vi "Voltage_demand.vi"() -> ()   [LabVIEW 2013]
uses:
  <vilib>/DAQmx/create/channels.llb/DAQmx Create Channel (CO-Pulse Generation-Frequency).vi
  <vilib>/DAQmx/configure/timing.llb/DAQmx Timing (Implicit).vi
panel:
  in  "stop vi":bool
  in  "counter":tag
  in  "stop blinking":bool
  in  "Blink":bool
  in  "Frequency [Hz]":dbl format="%#_3p"
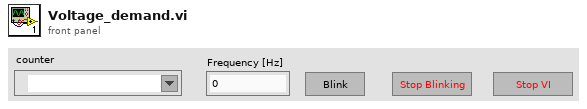
[diagram p1: front panel]
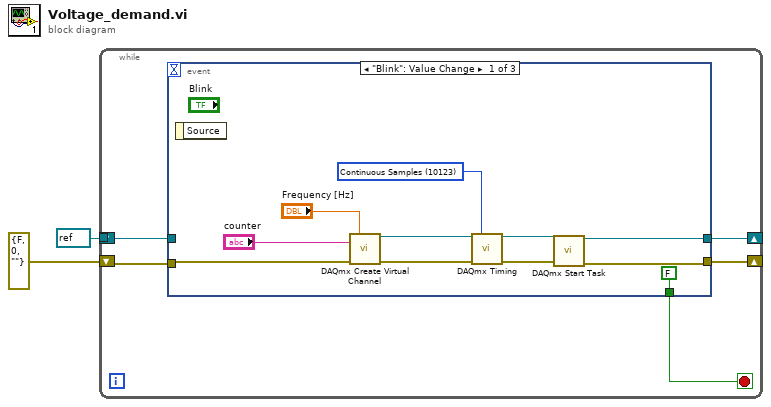
[diagram p0: block diagram]
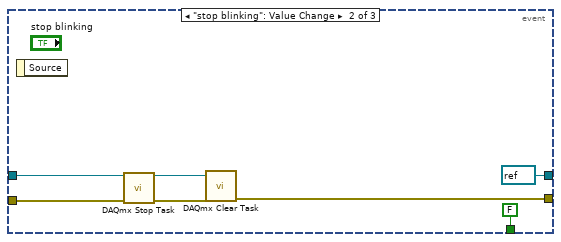
[diagram p2: hidden frame]
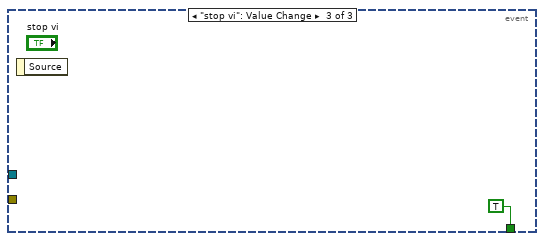
[diagram p3: hidden frame]
diagram:
  n1 = while {
    shift-right: [w6] -> _
    shift-left: refnum<k21> refnum ("task out") -> [w7]
    tunnel: [w7] -> _
    shift-right: [w4] -> _
    shift-left: errorcluster {"status"=FALSE, "code"=0, "source"=""} ("error out") -> [w5]
    stop <- w3 stop-if-true
    n2 = event shown="[0] \"Blink\": Value Change" {
      selector: _ -> [_ _ _]
      dyn-events: _ -> [_ _ _]
      timeout: _ -> [_ _ _]
      tunnel: [w11 refnum<k21> refnum ("task out") _] -> w6
      tunnel: w7 -> [_ w25 _]
      tunnel: w5 -> [w10 w23 _]
      tunnel: [w9 w22 _] -> w4
      tunnel: [FALSE FALSE TRUE] -> w3
      event "Blink": Value Change {
        w14 = 10123 items=["Finite Samples"=10178, "Continuous Samples"=10123, "Hardware Timed Single Point"=12522] ("sample mode")
        n3 = event-data() -> ()  [unwired: 1 in, 1 out]
        n4 = call-poly <vilib>:"DAQmx Create Virtual Channel.vi"("frequency"="Frequency [Hz]", "counter"="counter", "error in"=w10) -> ("task out"=w16:refnum<k21>, "error out"=w15:errorcluster)  [unwired: 11 in]
        n5 = call-poly <vilib>:"DAQmx Timing.vi"("task/channels in"=w16, "sample mode"=w14, "error in"=w15) -> ("task out"=w13:refnum<k21>, "error out"=w12:errorcluster)  [unwired: 11 in]
        n6 = call <vilib>:"DAQmx Start Task.vi"("task/channels in"=w13, "error in"=w12) -> ("task out"=w11:refnum<k21>, "error out"=w9:errorcluster)  [unwired: 12 in]
      }
      event "stop blinking": Value Change {
        n7 = event-data() -> ()  [unwired: 1 in, 1 out]
        n8 = call <vilib>:"DAQmx Stop Task.vi"("task/channels in"=w25, "error in"=w23) -> ("task out"=w24:refnum<k21>, "error out"=w21:errorcluster)  [unwired: 12 in]
        n9 = call <vilib>:"DAQmx Clear Task.vi"("task in"=w24, "error in"=w21) -> ("error out"=w22:errorcluster)  [unwired: 13 in]
      }
      event "stop vi": Value Change {
        n10 = event-data() -> ()  [unwired: 1 in, 1 out]
      }
    }
  }
